vi "Test Code 2.vi"   [LabVIEW 2023]
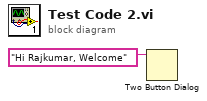
[diagram p0: block diagram]
diagram:
  n1 = Two Button Dialog(message="Hi Rajkumar, Welcome") -> ()  [unwired: 2 in, 1 out]
